vi "Destructor.vi"(8 "error in":errorcluster, 11 "RealMeasureLimit":refnum<class "RealMeasureLimit.lvclass">) -> (0 "error out":errorcluster)   [LabVIEW 2021, in "ProligentXMLGenerator.lvlib" / "RealMeasureLimit.lvclass"]
uses:
  RealMeasureLimit.lvclass
  RealMeasureLimit.lvclass/RealMeasureLimit.ctl
  MeasureLimit/MeasureLimit.lvclass
  RangeMeasureLimit/RangeMeasureLimit.lvclass
  C:/Projects/proligent-xml-generator-labview/src/ProligentXMLGenerator/Measure/RangeMeasureLimit/RangeMeasureLimit.lvclass
  C:/Projects/proligent-xml-generator-labview/src/ProligentXMLGenerator/Measure/MeasureLimit/MeasureLimit.lvclass
  C:/Projects/proligent-xml-generator-labview/src/ProligentXMLGenerator/Measure/RealMeasureLimit/RealMeasureLimit.lvclass
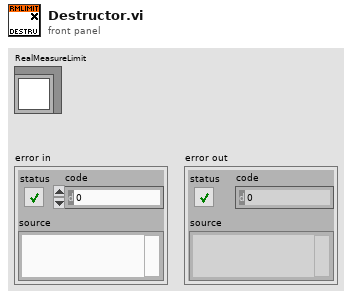
[diagram p1: front panel]
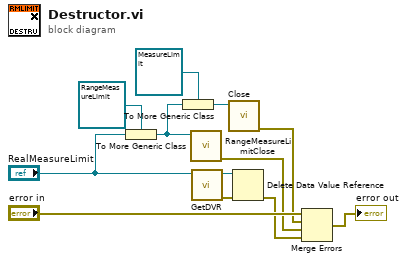
[diagram p0: block diagram]
diagram:
  n1 = To More Generic Class(target class=refnum<class "RangeMeasureLimit.lvclass"> refnum ("ProligentResultProcessor:RangeMeasureLimit"), reference="RealMeasureLimit") -> (generic class reference=w1:refnum<class "RangeMeasureLimit.lvclass">)
  n2 = To More Generic Class(target class=refnum<class "MeasureLimit.lvclass"> refnum ("ProligentResultProcessor:MeasureLimit"), reference=w1) -> (generic class reference=w2:refnum<class "MeasureLimit.lvclass">)
  n3 = call "RangeMeasureLimitClose.vi"("RangeMeasureLimit"=w1) -> ("error out"=w5:errorcluster)  [unwired: 10 in]
  n4 = call "GetDVR.vi"("RealMeasureLimit"="RealMeasureLimit") -> ("error out"=w9:errorcluster, "DVRReference"=w10:refnum<data-value>)  [unwired: 9 in]
  n5 = call "Close.vi"("MeasureLimit"=w2) -> ("error out"=w8:errorcluster)  [unwired: 10 in]
  n6 = Delete Data Value Reference(data value reference=w10, error in=w9) -> (error out=w7:errorcluster)  [unwired: 1 out]
  n7 = Merge Errors("error in", w8, w5, w7) -> (→"error out":errorcluster)
